vi "GVmotor_get_status.vi"(8 "error in":errorcluster, 10 "milliseconds to wait":u32=100, 11 "VISA in":refnum<visa-resource-name>) -> (0 "error out":errorcluster, 2 "Status Code":i32, 3 "VISA out":refnum<visa-resource-name>)   [LabVIEW 2019]
panel:
  out "trimmed string":string
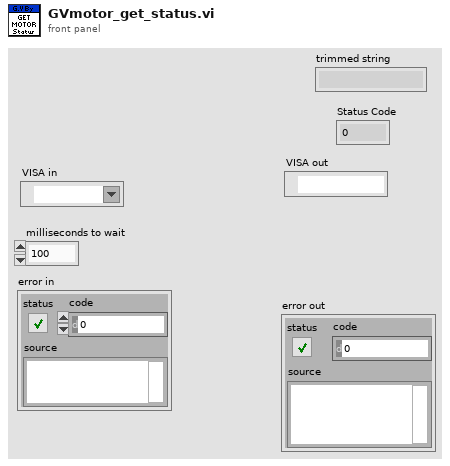
[diagram p1: front panel]
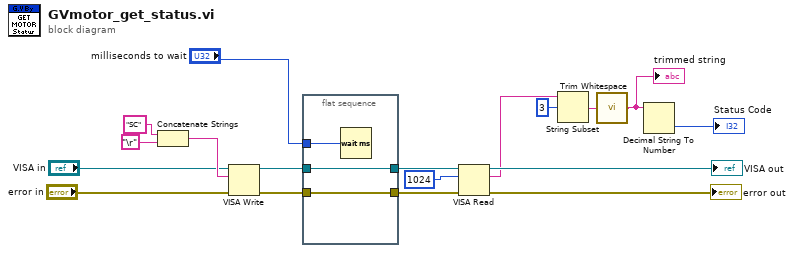
[diagram p0: block diagram]
diagram:
  n1 = Concatenate Strings("SC" ("string"), "\r") -> (w18:string)
  n2 = VISA Write(VISA resource name="VISA in", write buffer=w18, error in (no error)="error in") -> (VISA resource name out=w14:refnum<visa-resource-name>, error out=w15:errorcluster)  [unwired: 1 out]
  n3 = flat-sequence {
    tunnel: [w21] -> w2
    tunnel: w15 -> [w21]
    tunnel: [w20] -> w13
    tunnel: w14 -> [w20]
    tunnel: "milliseconds to wait" -> [w19]
    frame #0 {
      n4 = Wait (ms)(milliseconds to wait=w19) -> ()  [unwired: 1 out]
    }
  }
  n5 = VISA Read(VISA resource name=w13, byte count=u32 1024, error in (no error)=w2) -> (VISA resource name out=→"VISA out":refnum<visa-resource-name>, read buffer=w7:string, error out=→"error out":errorcluster)  [unwired: 1 out]
  n6 = String Subset(string=w7, offset (0)=3) -> (substring=w5:string)  [unwired: 1 in]
  n7 = call <vilib>:"Trim Whitespace.vi"("string"=w5) -> ("trimmed string"=w4:string)  [unwired: 1 in]
  "trimmed string" <- w4
  n8 = Decimal String To Number(string=w4) -> (number=→"Status Code":i32)  [unwired: 2 in, 1 out]
